vi "from string.vi"(8 "error in":errorcluster, 9 "data":string, 10 "version":string, 11 "TDMS datalogger configuration in":refnum<class "TDMS datalogger configuration.lvclass">) -> (0 "error out":errorcluster, 3 "TDMS datalogger configuration out":refnum<class "TDMS datalogger configuration.lvclass">)   [LabVIEW 2015, in "TDMS datalogger configuration.lvclass"]
doc: "Provides an interface for loading a module configuration from a file or other serialized data source. It is recommended that all children of this class store data in two sets--data required for its own initialization, and any data required for parent initialization--and that each implementation uses the <b>Call Parent Method</b> primitive to de-serialize parent information. As a result, it is expected that every module configuration class calls <b>component configuration.lvclass:From String.vi</b>."
uses:
  TDMS datalogger configuration.lvclass
  <vilib>/NI/Tag Bus Module Framework/channel/TBM channel.lvclass
  <vilib>/NI/LogRotate/options.ctl
  Logging Type.ctl
  Trigger Type.ctl
  Edge Direction.ctl
  TDMS datalogger configuration.lvclass/TDMS datalogger configuration.ctl
  <vilib>/NI/Tag Bus Module Framework/module configuration/TBM module configuration.lvclass
  <vilib>/NI/Configuration Framework/serializable configuration/NISE_CEF_serializable configuration.lvclass
  <vilib>/NI/LogRotate/LogRotate.lvclass
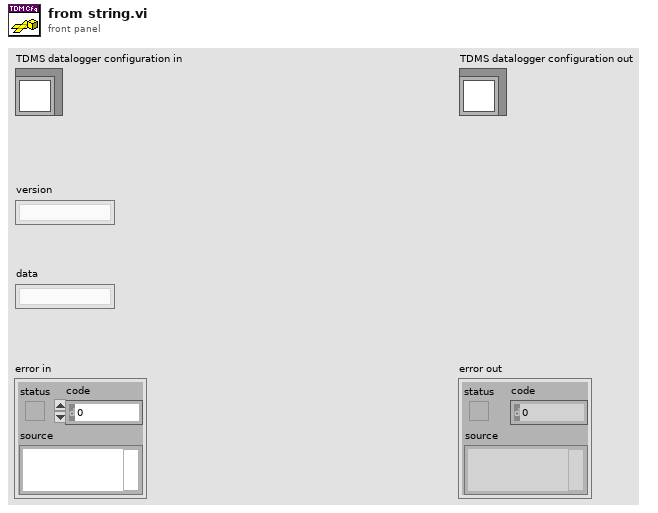
[diagram p1: front panel]
types:
  T1 = typedef "TDMS datalogger configuration.lvclass/Edge Direction.ctl" = enum16{"Rising", "Falling"}
  T2 = typedef "TDMS datalogger configuration.lvclass/Trigger Type.ctl" = enum16{"None", "Start"}
  T3 = typedef "TDMS datalogger configuration.lvclass/Logging Type.ctl" = enum16{"Continuous", "Finite"}
  T4 = typedef "LogRotate.lvclass/options.ctl" = cluster{"max file size (bytes)":i64, "rotate count":u32, "max age (days)":dbl, "No archive dir":bool, "Archive dir":path}
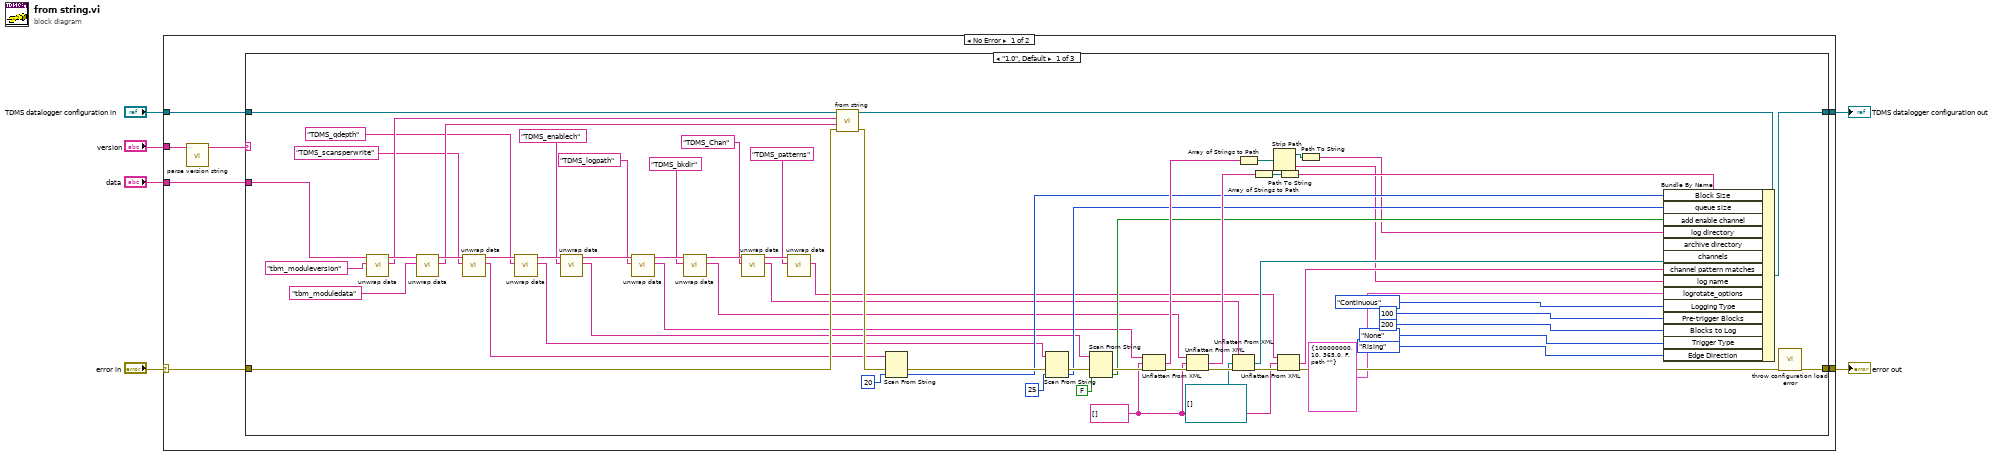
[diagram p0: block diagram]
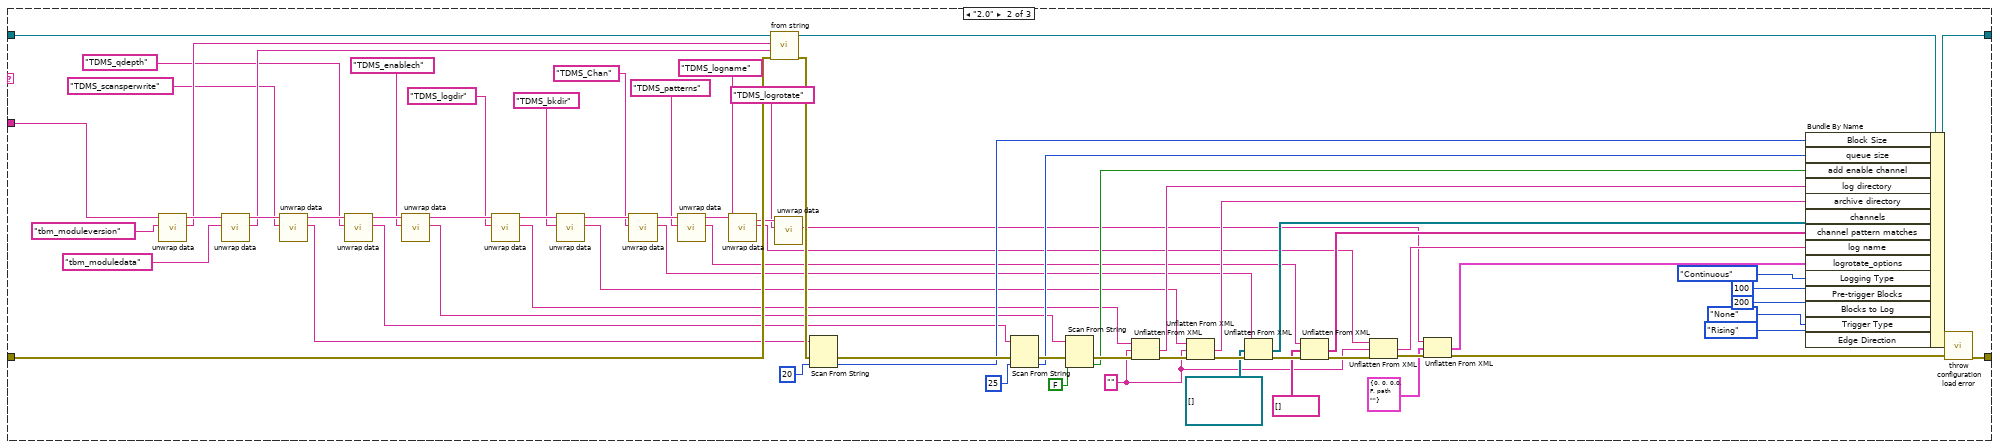
[diagram p2: hidden frame]
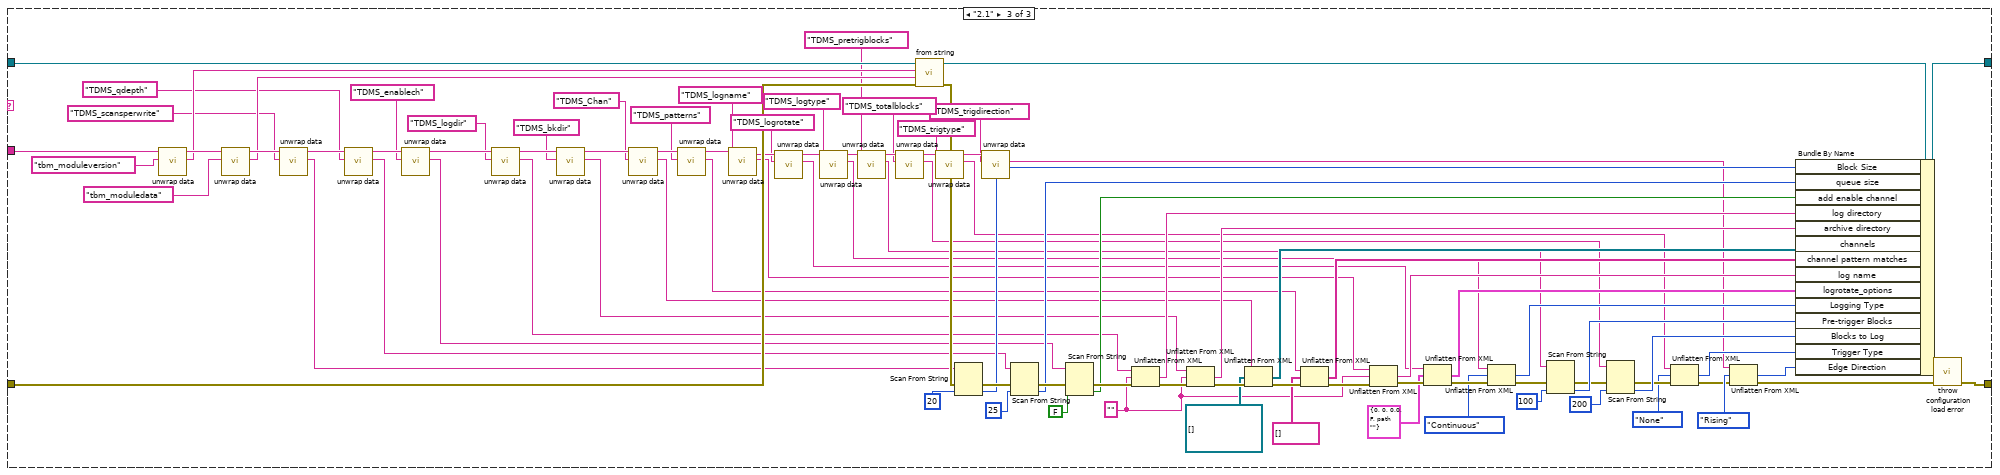
[diagram p3: hidden frame]
diagram:
  n1 = case shown="No Error" "error in" {
    selector: "error in" -> [w7 w242]
    tunnel: "data" -> [w13 _]
    tunnel: "TDMS datalogger configuration in" -> [w12 w241]
    tunnel: [w11 w241] -> w5
    tunnel: [w10 w242] -> w4
    tunnel: "version" -> [w9 _]
    frame No Error {
      n2 = call <vilib>:"parse version string.vi"("full version"=w9) -> ("major.minor version"=w8:string)  [unwired: 7 in, 3 out]
      n3 = case shown="\"1.0\", Default" w8 {
        tunnel: w13 -> [w60 w129 w223]
        tunnel: w7 -> [w74 w143 w237]
        tunnel: w12 -> [w77 w146 w240]
        tunnel: [w76 w145 w239] -> w11
        tunnel: [w33 w102 w196] -> w10
        frame "1.0", Default {
          w28 = string[] [] ("array of strings")
          n4 = call <vilib>:"unwrap data.vi"("identifier"="tbm_moduleversion" ("additional identifier"), "data to unwrap"=w60) -> ("unwrapped data"=w59:string, "remaining string"=w66:string)  [unwired: 8 in]
          n5 = call <vilib>:"unwrap data.vi"("identifier"="tbm_moduledata" ("additional identifier"), "data to unwrap"=w66) -> ("unwrapped data"=w58:string, "remaining string"=w63:string)  [unwired: 8 in]
          n6 = call <vilib>:"unwrap data.vi"("identifier"="TDMS_scansperwrite" ("additional identifier"), "data to unwrap"=w63) -> ("unwrapped data"=w44:string, "remaining string"=w62:string)  [unwired: 8 in]
          n7 = call <vilib>:"unwrap data.vi"("identifier"="TDMS_qdepth" ("additional identifier"), "data to unwrap"=w62) -> ("unwrapped data"=w42:string, "remaining string"=w61:string)  [unwired: 8 in]
          n8 = call <vilib>:"unwrap data.vi"("identifier"="TDMS_enablech" ("additional identifier"), "data to unwrap"=w61) -> ("unwrapped data"=w40:string, "remaining string"=w48:string)  [unwired: 8 in]
          n9 = call <vilib>:"unwrap data.vi"("identifier"="TDMS_logpath" ("additional identifier"), "data to unwrap"=w48) -> ("unwrapped data"=w38:string, "remaining string"=w47:string)  [unwired: 8 in]
          n10 = call <vilib>:"unwrap data.vi"("identifier"="TDMS_bkdir" ("additional identifier"), "data to unwrap"=w47) -> ("unwrapped data"=w37:string, "remaining string"=w46:string)  [unwired: 8 in]
          n11 = call <vilib>:"unwrap data.vi"("identifier"="TDMS_Chan" ("additional identifier"), "data to unwrap"=w46) -> ("unwrapped data"=w36:string, "remaining string"=w32:string)  [unwired: 8 in]
          n12 = call <vilib>:"unwrap data.vi"("identifier"="TDMS_patterns", "data to unwrap"=w32) -> ("unwrapped data"=w27:string)  [unwired: 8 in, 1 out]
          n13 = call-parent "from string.vi"("error in"=w74, "data"=w58, "version"=w59, "module configuration in"=w77) -> ("error out"=w75:errorcluster, "module configuration out"=w73:refnum<class "TDMS datalogger configuration.lvclass">)  [unwired: 6 in]
          n14 = Scan From String(input string=w44, error in=w75, default 1=u16 20 ("scans per write")) -> (error out=w55:errorcluster, output 1=w49:u16)  [unwired: 2 in, 2 out]
          n15 = Scan From String(input string=w42, error in=w55, default 1=u16 25 ("queue size")) -> (error out=w56:errorcluster, output 1=w51:u16)  [unwired: 2 in, 2 out]
          n16 = Scan From String(input string=w40, error in=w56, default 1=FALSE ("add enable channel")) -> (error out=w57:errorcluster, output 1=w53:bool)  [unwired: 2 in, 2 out]
          n17 = Unflatten From XML(xml string=w38, type=w28, error in (no error)=w57) -> (value=w67:string[], error out=w71:errorcluster)
          n18 = Unflatten From XML(xml string=w37, type=w28, error in (no error)=w71) -> (value=w68:string[], error out=w72:errorcluster)
          n19 = Unflatten From XML(xml string=w36, type=refnum<class "TBM channel.lvclass">[] [] ("channels"), error in (no error)=w72) -> (value=w69:refnum<class "TBM channel.lvclass">[], error out=w30:errorcluster)
          n20 = Array of Strings to Path(0:w67) -> (2:w23:path)  [unwired: 1 in]
          n21 = Array of Strings to Path(0:w68) -> (2:w25:path)  [unwired: 1 in]
          n22 = Strip Path(path=w23) -> (stripped path=w21:path, name=w22:string)
          n23 = Unflatten From XML(xml string=w27, type=w28, error in (no error)=w30) -> (value=w26:string[], error out=w29:errorcluster)
          n24 = Path To String(path=w25) -> (string=w24:string)
          n25 = Path To String(path=w21) -> (string=w20:string)
          n26 = Bundle By Name(cluster=w73, "Block Size"=w49, "queue size"=w51, "add enable channel"=w53, "log directory"=w20, "archive directory"=w24, "channels"=w69, "channel pattern matches"=w26, "log name"=w22, "logrotate_options"=T4 {"max file size (bytes)"=100000000, "rotate count"=10, "max age (days)"=365.0, "No archive dir"=FALSE, "Archive dir"=path ""}, "Logging Type"=Logging_Type."Continuous", "Pre-trigger Blocks"=100, "Blocks to Log"=200, "Trigger Type"=Trigger_Type."None", "Edge Direction"=Edge_Direction."Rising") -> (w76:refnum<class "TDMS datalogger configuration.lvclass">)
          n27 = call <vilib>:"throw configuration load error.vi"("error in"=w29) -> ("error out"=w33:errorcluster)  [unwired: 10 in]
        }
        frame "2.0" {
          w94 = ""
          n28 = call <vilib>:"unwrap data.vi"("identifier"="tbm_moduleversion" ("additional identifier"), "data to unwrap"=w129) -> ("unwrapped data"=w128:string, "remaining string"=w135:string)  [unwired: 8 in]
          n29 = call <vilib>:"unwrap data.vi"("identifier"="tbm_moduledata" ("additional identifier"), "data to unwrap"=w135) -> ("unwrapped data"=w127:string, "remaining string"=w132:string)  [unwired: 8 in]
          n30 = call <vilib>:"unwrap data.vi"("identifier"="TDMS_scansperwrite" ("additional identifier"), "data to unwrap"=w132) -> ("unwrapped data"=w113:string, "remaining string"=w131:string)  [unwired: 8 in]
          n31 = call <vilib>:"unwrap data.vi"("identifier"="TDMS_qdepth" ("additional identifier"), "data to unwrap"=w131) -> ("unwrapped data"=w111:string, "remaining string"=w130:string)  [unwired: 8 in]
          n32 = call <vilib>:"unwrap data.vi"("identifier"="TDMS_enablech" ("additional identifier"), "data to unwrap"=w130) -> ("unwrapped data"=w109:string, "remaining string"=w117:string)  [unwired: 8 in]
          n33 = call <vilib>:"unwrap data.vi"("identifier"="TDMS_logdir" ("additional identifier"), "data to unwrap"=w117) -> ("unwrapped data"=w107:string, "remaining string"=w116:string)  [unwired: 8 in]
          n34 = call <vilib>:"unwrap data.vi"("identifier"="TDMS_bkdir" ("additional identifier"), "data to unwrap"=w116) -> ("unwrapped data"=w106:string, "remaining string"=w115:string)  [unwired: 8 in]
          n35 = call <vilib>:"unwrap data.vi"("identifier"="TDMS_Chan" ("additional identifier"), "data to unwrap"=w115) -> ("unwrapped data"=w105:string, "remaining string"=w101:string)  [unwired: 8 in]
          n36 = call <vilib>:"unwrap data.vi"("identifier"="TDMS_patterns", "data to unwrap"=w101) -> ("unwrapped data"=w97:string, "remaining string"=w92:string)  [unwired: 8 in]
          n37 = call <vilib>:"unwrap data.vi"("identifier"="TDMS_logname", "data to unwrap"=w92) -> ("unwrapped data"=w91:string, "remaining string"=w89:string)  [unwired: 8 in]
          n38 = call-parent "from string.vi"("error in"=w143, "data"=w127, "version"=w128, "module configuration in"=w146) -> ("error out"=w144:errorcluster, "module configuration out"=w142:refnum<class "TDMS datalogger configuration.lvclass">)  [unwired: 6 in]
          n39 = call <vilib>:"unwrap data.vi"("identifier"="TDMS_logrotate", "data to unwrap"=w89) -> ("unwrapped data"=w85:string)  [unwired: 8 in, 1 out]
          n40 = Scan From String(input string=w113, error in=w144, default 1=u16 20 ("scans per write")) -> (error out=w124:errorcluster, output 1=w118:u16)  [unwired: 2 in, 2 out]
          n41 = Scan From String(input string=w111, error in=w124, default 1=u16 25 ("queue size")) -> (error out=w125:errorcluster, output 1=w120:u16)  [unwired: 2 in, 2 out]
          n42 = Scan From String(input string=w109, error in=w125, default 1=FALSE ("add enable channel")) -> (error out=w126:errorcluster, output 1=w122:bool)  [unwired: 2 in, 2 out]
          n43 = Unflatten From XML(xml string=w107, type=w94, error in (no error)=w126) -> (value=w136:string, error out=w140:errorcluster)
          n44 = Unflatten From XML(xml string=w106, type=w94, error in (no error)=w140) -> (value=w137:string, error out=w141:errorcluster)
          n45 = Unflatten From XML(xml string=w105, type=refnum<class "TBM channel.lvclass">[] [] ("channels"), error in (no error)=w141) -> (value=w138:refnum<class "TBM channel.lvclass">[], error out=w99:errorcluster)
          n46 = Unflatten From XML(xml string=w97, type=string[] [] ("array of strings"), error in (no error)=w99) -> (value=w96:string[], error out=w95:errorcluster)
          n47 = Unflatten From XML(xml string=w91, type=w94, error in (no error)=w95) -> (value=w93:string, error out=w87:errorcluster)
          n48 = Unflatten From XML(xml string=w85, type=T4 {"max file size (bytes)"=0, "rotate count"=0, "max age (days)"=0.0, "No archive dir"=FALSE, "Archive dir"=path ""} ("logrotate_options"), error in (no error)=w87) -> (value=w83:T4, error out=w86:errorcluster)
          n49 = Bundle By Name(cluster=w142, "Block Size"=w118, "queue size"=w120, "add enable channel"=w122, "log directory"=w136, "archive directory"=w137, "channels"=w138, "channel pattern matches"=w96, "log name"=w93, "logrotate_options"=w83, "Logging Type"=Logging_Type."Continuous", "Pre-trigger Blocks"=100, "Blocks to Log"=200, "Trigger Type"=Trigger_Type."None", "Edge Direction"=Edge_Direction."Rising") -> (w145:refnum<class "TDMS datalogger configuration.lvclass">)
          n50 = call <vilib>:"throw configuration load error.vi"("error in"=w86) -> ("error out"=w102:errorcluster)  [unwired: 10 in]
        }
        frame "2.1" {
          w188 = ""
          n51 = call <vilib>:"unwrap data.vi"("identifier"="tbm_moduleversion" ("additional identifier"), "data to unwrap"=w223) -> ("unwrapped data"=w222:string, "remaining string"=w229:string)  [unwired: 8 in]
          n52 = call <vilib>:"unwrap data.vi"("identifier"="tbm_moduledata" ("additional identifier"), "data to unwrap"=w229) -> ("unwrapped data"=w221:string, "remaining string"=w226:string)  [unwired: 8 in]
          n53 = call <vilib>:"unwrap data.vi"("identifier"="TDMS_scansperwrite" ("additional identifier"), "data to unwrap"=w226) -> ("unwrapped data"=w207:string, "remaining string"=w225:string)  [unwired: 8 in]
          n54 = call <vilib>:"unwrap data.vi"("identifier"="TDMS_qdepth" ("additional identifier"), "data to unwrap"=w225) -> ("unwrapped data"=w205:string, "remaining string"=w224:string)  [unwired: 8 in]
          n55 = call <vilib>:"unwrap data.vi"("identifier"="TDMS_enablech" ("additional identifier"), "data to unwrap"=w224) -> ("unwrapped data"=w203:string, "remaining string"=w211:string)  [unwired: 8 in]
          n56 = call <vilib>:"unwrap data.vi"("identifier"="TDMS_logdir" ("additional identifier"), "data to unwrap"=w211) -> ("unwrapped data"=w201:string, "remaining string"=w210:string)  [unwired: 8 in]
          n57 = call <vilib>:"unwrap data.vi"("identifier"="TDMS_bkdir" ("additional identifier"), "data to unwrap"=w210) -> ("unwrapped data"=w200:string, "remaining string"=w209:string)  [unwired: 8 in]
          n58 = call <vilib>:"unwrap data.vi"("identifier"="TDMS_Chan" ("additional identifier"), "data to unwrap"=w209) -> ("unwrapped data"=w199:string, "remaining string"=w195:string)  [unwired: 8 in]
          n59 = call <vilib>:"unwrap data.vi"("identifier"="TDMS_patterns", "data to unwrap"=w195) -> ("unwrapped data"=w191:string, "remaining string"=w186:string)  [unwired: 8 in]
          n60 = call <vilib>:"unwrap data.vi"("identifier"="TDMS_logname", "data to unwrap"=w186) -> ("unwrapped data"=w185:string, "remaining string"=w183:string)  [unwired: 8 in]
          n61 = call <vilib>:"unwrap data.vi"("identifier"="TDMS_logrotate", "data to unwrap"=w183) -> ("unwrapped data"=w180:string, "remaining string"=w161:string)  [unwired: 8 in]
          n62 = call <vilib>:"unwrap data.vi"("identifier"="TDMS_logtype", "data to unwrap"=w161) -> ("unwrapped data"=w155:string, "remaining string"=w160:string)  [unwired: 8 in]
          n63 = call <vilib>:"unwrap data.vi"("identifier"="TDMS_pretrigblocks", "data to unwrap"=w160) -> ("unwrapped data"=w154:string, "remaining string"=w159:string)  [unwired: 8 in]
          n64 = call <vilib>:"unwrap data.vi"("identifier"="TDMS_totalblocks", "data to unwrap"=w159) -> ("unwrapped data"=w153:string, "remaining string"=w158:string)  [unwired: 8 in]
          n65 = call-parent "from string.vi"("error in"=w237, "data"=w221, "version"=w222, "module configuration in"=w240) -> ("error out"=w238:errorcluster, "module configuration out"=w236:refnum<class "TDMS datalogger configuration.lvclass">)  [unwired: 6 in]
          n66 = call <vilib>:"unwrap data.vi"("identifier"="TDMS_trigtype", "data to unwrap"=w158) -> ("unwrapped data"=w152:string, "remaining string"=w157:string)  [unwired: 8 in]
          n67 = Scan From String(input string=w207, error in=w238, default 1=u16 20 ("scans per write")) -> (error out=w218:errorcluster, output 1=w212:u16)  [unwired: 2 in, 2 out]
          n68 = call <vilib>:"unwrap data.vi"("identifier"="TDMS_trigdirection", "data to unwrap"=w157) -> ("unwrapped data"=w156:string)  [unwired: 8 in, 1 out]
          n69 = Scan From String(input string=w205, error in=w218, default 1=u16 25 ("queue size")) -> (error out=w219:errorcluster, output 1=w214:u16)  [unwired: 2 in, 2 out]
          n70 = Scan From String(input string=w203, error in=w219, default 1=FALSE ("add enable channel")) -> (error out=w220:errorcluster, output 1=w216:bool)  [unwired: 2 in, 2 out]
          n71 = Unflatten From XML(xml string=w201, type=w188, error in (no error)=w220) -> (value=w230:string, error out=w234:errorcluster)
          n72 = Unflatten From XML(xml string=w200, type=w188, error in (no error)=w234) -> (value=w231:string, error out=w235:errorcluster)
          n73 = Unflatten From XML(xml string=w199, type=refnum<class "TBM channel.lvclass">[] [] ("channels"), error in (no error)=w235) -> (value=w232:refnum<class "TBM channel.lvclass">[], error out=w193:errorcluster)
          n74 = Unflatten From XML(xml string=w191, type=string[] [] ("array of strings"), error in (no error)=w193) -> (value=w190:string[], error out=w189:errorcluster)
          n75 = Unflatten From XML(xml string=w185, type=w188, error in (no error)=w189) -> (value=w187:string, error out=w181:errorcluster)
          n76 = Unflatten From XML(xml string=w180, type=T4 {"max file size (bytes)"=0, "rotate count"=0, "max age (days)"=0.0, "No archive dir"=FALSE, "Archive dir"=path ""} ("logrotate_options"), error in (no error)=w181) -> (value=w178:T4, error out=w177:errorcluster)
          n77 = Unflatten From XML(xml string=w155, type=Logging_Type."Continuous" ("Logging Type"), error in (no error)=w177) -> (value=w175:T3, error out=w174:errorcluster)
          n78 = Scan From String(input string=w154, error in=w174, default 1=100 ("default value 1")) -> (error out=w171:errorcluster, output 1=w172:i32)  [unwired: 2 in, 2 out]
          n79 = Scan From String(input string=w153, error in=w171, default 1=200 ("default value 1")) -> (error out=w168:errorcluster, output 1=w169:i32)  [unwired: 2 in, 2 out]
          n80 = Unflatten From XML(xml string=w152, type=Trigger_Type."None" ("Trigger Type"), error in (no error)=w168) -> (value=w166:T2, error out=w164:errorcluster)
          n81 = Unflatten From XML(xml string=w156, type=Edge_Direction."Rising" ("Edge Direction"), error in (no error)=w164) -> (value=w163:T1, error out=w162:errorcluster)
          n82 = Bundle By Name(cluster=w236, "Block Size"=w212, "queue size"=w214, "add enable channel"=w216, "log directory"=w230, "archive directory"=w231, "channels"=w232, "channel pattern matches"=w190, "log name"=w187, "logrotate_options"=w178, "Logging Type"=w175, "Pre-trigger Blocks"=w172, "Blocks to Log"=w169, "Trigger Type"=w166, "Edge Direction"=w163) -> (w239:refnum<class "TDMS datalogger configuration.lvclass">)
          n83 = call <vilib>:"throw configuration load error.vi"("error in"=w162) -> ("error out"=w196:errorcluster)  [unwired: 10 in]
        }
      }
    }
    frame Error {
    }
  }
  "error out" <- w4
  "TDMS datalogger configuration out" <- w5
